vi "_GainComp_LockInAmp_2.vi"(9 "GC_LockinAmp":T3={"GPIB"="28", "wait(s)"=10.0, "measure(s) "=30.0, "save"=FALSE, "time constant"=6, "file_name"=""} {"time constant" items=["100mS"=5, "300mS"=6, "1S"=7, "3S"=8, "10S"=9]}, 10 "Control":T4={"GPIB_ATT"="28", "6501Dev#"=1, "GPIB_SP"="18", "GPIB_PM"="13", "GPIB_DSA"="11", "GPIB_DMM (TPD)"="23", "GPIB_MPI"="COM5", "mortor設定"=[{"Axis"=0, "ID"=0, "HIspeed"=200.0, "LOspeed"=100.0, "ACCEL(ms)"=100.0, "Sratio"=50.0, "フリーラン\n"=FALSE, "文字列"="DSB HOT/COLD"}, {"Axis"=1, "ID"=0, "HIspeed"=4.0, "LOspeed"=4.0, "ACCEL(ms)"=100.0, "Sratio"=50.0, "フリーラン\n"=TRUE, "文字列"="SubMM Att"}, {"Axis"=0, "ID"=0, "HIspeed"=200.0, "LOspeed"=100.0, "ACCEL(ms)"=100.0, "Sratio"=50.0, "フリーラン\n"=FALSE, "文字列"="MPI Port1"}, {"Axis"=1, "ID"=0, "HIspeed"=200.0, "LOspeed"=100.0, "ACCEL(ms)"=100.0, "Sratio"=50.0, "フリーラン\n"=FALSE, "文字列"="MPI Port2"}, {"Axis"=1, "ID"=0, "HIspeed"=200.0, "LOspeed"=100.0, "ACCEL(ms)"=100.0, "Sratio"=50.0, "フリーラン\n"=TRUE, "文字列"="gainComp"}], "DATAパス"=path "C:/Documents and Settings/band10/デスクトップ/data/cartridge/CCA03/CCA-03-13/110629_SBR_P1", "DBパス "=path "Z:/band10/Labview_ALMA/MIX95/test", "comment"="110629_SBR_P1", "ColdCarts"="003601", "Th"=299.0, "Tc"=83.0, "Set_SIS_volt"=2.1, "Offset"=0.0, "control"=0, "FreqLO"=874.0, "Set_Mag_Cur"=8.86861313868613, "MPI offset(mm)"=23.166, "HOT/COLD"=1} {"HOT/COLD" items=["DSB", "SBR (Cart.)", "GainComp", "SBR (MIX)"]; "control" items=["CLOSE LOOP", "OPEN LOOP", "Not Control"]}, 11 "Bias_LO_equip":T1={"Node address"=19, "CAN Interface"="CAN0", "Cartridge band"=10, "Slave Node in"={"Address"=19, "Serial Number"=[16, -88, -112, 75, 1, 8, 0, 24]}, "ObjHandle out"=93257792, "POL"=0, "sb"=1, "GPIB_SM (SIS S,V)"="24", "GPIB_DMM (SIS I)"="22", "GPIB_SM (MAG I) "="25", "GPIB_SG(LO)"="19", "GPIB_PW (PAMP) "="6", "GPIB_TMP1(8ch)"="12", "GPIB_TMP2(2ch)  "="13", "WCA_avg"=10, "Rsen"=10.0, "BiasModule"=1, "LOModule "=2, "WCA_LO_FREQ_SET"={"YTO Low freq. [GHz]"=14.66, "YTO High freq. [GHz]"=17.5, "Kvco"=1, "Lock Pol."=0, "SET LO FREQ"=97.111115, "Multiplier"=6.0, "YTO (HEX)"=2196, "YTO ( FREQ)"=16.18299, "NULL PLL INTEGRATOR"=FALSE}, "Res for"=0} {"Res for" items=["none", "series res", "parallel res"]; "WCA_LO_FREQ_SET"."YTO ( FREQ)" min=25 max=150 step=0.0001 format="%.3f"; "WCA_LO_FREQ_SET"."Multiplier" min=3 max=6 step=3; "WCA_LO_FREQ_SET"."SET LO FREQ" min=25 max=150 step=0.0001 format="%.3f"; "WCA_LO_FREQ_SET"."Lock Pol." items=["Lower", "Upper"]; "WCA_LO_FREQ_SET"."Kvco" items=["7.5MHz/V", "15MHz/V"]; "WCA_LO_FREQ_SET"."YTO High freq. [GHz]" format="%.3f"; "WCA_LO_FREQ_SET"."YTO Low freq. [GHz]" format="%.3f"; "LOModule" items=["Manual Gunn+PAMP"=0, "PLL GUNN+PAMP"=5, "B10Lab LO"=1, "WCA LO"=2, ""=3, "YIG発信器"=4, "none"=99]; "BiasModule" items=["B10Lab Bias"=0, "WCA BiasModule"=1, "none"=99]; "Slave Node in"."Serial Number" format="%.0x"; "Slave Node in"."Address" format="%.0x"; "Cartridge band" max=10 step=1; "Node address" format="%.0x"}) -> (3 "出力文字列":string="GainComp, 2011-02-04  14:13:24, 874.00,1, 0, 0.95,, 2.256E-3, 2.227E-3, 5.462E-6, 1.285E+0, 9.323E-1")   [LabVIEW 2017]
uses:
  <vilib>/Analysis/NI_AALBase.lvlib
panel:
  out "測定回数":dbl
  out "Ｖｃ　σ":bool
  out "Vh σ":bool
  out "Vh":bool
  out "Vc":bool
  out "TC":dbl=300.0
  out "ΔVh":dbl=4.302325581394609e-07 format="%#_6p"
  out "ΔVc":dbl=3.139534883720742e-07 format="%#_6p"
  out "GCls  2":dbl=0.08160280378442007 format="%#_6f"
  out "Error 2":dbl=0.0005369243568017377 format="%#_6f"
  out "GCdiff 2":dbl=-0.044394897546439334 format="%#_6f"
  out "Error 1":dbl=0.000518990604292761 format="%#_4f"
  out "GCls  1":dbl=0.12198673439194854 format="%#_4f"
  out "GCdiff 1":dbl=0.018739520662782047 format="%#_4f"
  out "Vh2 σ":dbl=2.8613203126074345e-06 format="%#_6p"
  out "Vh2":dbl=0.0011791627906976743 format="%#_6p"
  out "Vc2 σ":dbl=2.5850430165789864e-06 format="%#_6p"
  out "Vc2":dbl=0.0011786395348837209 format="%#_6p"
  out "AP":dbl[](array[numeric])
  out "AR":dbl[](array[numeric])
  out "AT":dbl[](array[numeric])
  out "Vh1 σ":dbl=2.507960747227626e-06 format="%#_6p"
  out "Vh1":dbl=0.0011787325581395349 format="%#_6p"
  out "Vc1 σ":dbl=1.671946233643571e-06 format="%#_6p"
  out "Vc1":dbl=0.001178953488372093 format="%#_6p"
  out "XYグラフ 2":cluster{dbl[], dbl[]}(graph)={[11.15625, 11.84375, 12.53125, 13.21875, 13.921875, 14.609375, 15.296875, 15.984375, 16.671875, 17.359375, 18.046875, 18.734375, 19.421875, 20.109375, 20.796875, 21.484375, 22.171875, 22.859375, 23.546875, 24.234375, 24.921875, 25.625, 26.3125, 27.0, 27.6875, 28.375, 29.0625, 29.75, 30.4375, 31.125, 31.8125, 32.5, 33.1875, 33.875, 34.5625, 35.25, 35.9375, 36.625, 37.3125, 38.0, 38.703125, 39.390625, 40.078125, 51.171875, 51.859375, 52.546875, 53.234375, 53.9375, 54.625, 55.3125, 56.0, 56.6875, 57.375, 58.0625, 58.75, 59.4375, 60.125, 60.8125, 61.5, 62.1875, 62.875, 63.5625, 64.25, 64.9375, 65.625, 66.328125, 67.015625, 67.703125, 68.390625, 69.078125, 69.765625, 70.453125, 71.140625, 71.828125, 72.515625, 73.203125, 73.890625, 74.578125, 75.265625, 75.953125, 76.640625, 77.328125, 78.015625, 78.71875, 79.40625, 80.09375, 91.203125, 91.890625, 92.578125, 93.265625, 93.953125, 94.640625, 95.328125, 96.015625, 96.703125, 97.390625, 98.078125, 98.765625, 99.453125, 100.140625, 100.828125, 101.515625, 102.203125, 102.890625, 103.59375, 104.28125, 104.96875, 105.65625, 106.34375, 107.03125, 107.71875, 108.40625, 109.09375, 109.78125, 110.46875, 111.15625, 111.84375, 112.53125, 113.21875, 113.90625, 114.59375, 115.28125, 115.984375, 116.671875, 117.359375, 118.046875, 118.734375, 119.421875, 120.109375, 131.203125, 131.890625, 132.578125, 133.265625, 133.953125, 134.65625, 135.34375, 136.03125, 136.71875, 137.40625, 138.09375, 138.78125, 139.46875, 140.15625, 140.84375, 141.53125, 142.21875, 142.90625, 143.59375, 144.28125, 144.96875, 145.65625, 146.34375, 147.03125, 147.734375, 148.421875, 149.109375, 149.796875, 150.484375, 151.171875, 151.859375, 152.546875, 153.234375, 153.921875, 154.609375, 155.296875, 155.984375, 156.671875, 157.359375, 158.046875, 158.734375, 159.4375, 160.125], [98.35, 97.45, 97.75, 98.25, 97.5, 97.55, 97.65, 98.1, 98.15, 98.05, 98.1, 97.95, 98.1, 98.15, 98.5, 98.6, 98.35, 97.95, 98.05, 98.4, 98.3, 98.15, 98.45, 98.0, 98.3, 97.95, 98.25, 97.85, 97.45, 97.75, 97.3, 97.1, 97.3, 97.2, 97.7, 98.1, 98.1, 97.85, 97.9, 98.15, 97.8, 97.8, 97.35, 97.9, 97.65, 98.05, 98.15, 98.05, 97.85, 97.9, 97.75, 98.3, 98.8, 98.7, 98.05, 98.2, 98.85, 97.75, 97.65, 97.85, 98.15, 98.75, 98.75, 98.2, 97.55, 97.05, 96.75, 96.45, 96.8, 97.4, 97.45, 97.75, 98.35, 98.25, 98.5, 98.9, 98.7, 98.55, 98.75, 98.25, 98.45, 98.7, 98.45, 98.1, 98.25, 98.1, 96.6, 96.95, 96.7, 96.55, 96.05, 96.3, 96.2, 96.15, 95.85, 96.7, 96.9, 97.15, 98.05, 98.0, 98.1, 97.8, 98.05, 97.95, 98.0, 98.45, 98.1, 98.25, 98.25, 98.4, 98.35, 98.2, 98.1, 97.9, 98.3, 98.45, 98.65, 98.6, 98.45, 97.95, 98.6, 98.35, 98.25, 98.25, 98.25, 98.05, 98.1, 98.45, 98.6, 98.75, 98.4, 98.3, 98.7, 99.2, 98.75, 98.35, 98.05, 97.6, 98.4, 98.45, 98.4, 98.65, 98.25, 97.8, 98.2, 98.95, 97.75, 98.4, 98.45, 98.2, 97.75, 97.75, 98.15, 97.05, 96.35, 96.2, 96.2, 96.2, 97.0, 96.5, 96.35, 96.55, 96.45, 96.95, 97.15, 97.65, 97.4, 97.45, 97.9, 97.6, 97.5, 97.5]}
  out "P":dbl=97.35 format="%#_4f"
  out "XYグラフ":cluster{dbl[], dbl[]}(graph)={[11.15625, 11.84375, 12.53125, 13.21875, 13.921875, 14.609375, 15.296875, 15.984375, 16.671875, 17.359375, 18.046875, 18.734375, 19.421875, 20.109375, 20.796875, 21.484375, 22.171875, 22.859375, 23.546875, 24.234375, 24.921875, 25.625, 26.3125, 27.0, 27.6875, 28.375, 29.0625, 29.75, 30.4375, 31.125, 31.8125, 32.5, 33.1875, 33.875, 34.5625, 35.25, 35.9375, 36.625, 37.3125, 38.0, 38.703125, 39.390625, 40.078125, 51.171875, 51.859375, 52.546875, 53.234375, 53.9375, 54.625, 55.3125, 56.0, 56.6875, 57.375, 58.0625, 58.75, 59.4375, 60.125, 60.8125, 61.5, 62.1875, 62.875, 63.5625, 64.25, 64.9375, 65.625, 66.328125, 67.015625, 67.703125, 68.390625, 69.078125, 69.765625, 70.453125, 71.140625, 71.828125, 72.515625, 73.203125, 73.890625, 74.578125, 75.265625, 75.953125, 76.640625, 77.328125, 78.015625, 78.71875, 79.40625, 80.09375, 91.203125, 91.890625, 92.578125, 93.265625, 93.953125, 94.640625, 95.328125, 96.015625, 96.703125, 97.390625, 98.078125, 98.765625, 99.453125, 100.140625, 100.828125, 101.515625, 102.203125, 102.890625, 103.59375, 104.28125, 104.96875, 105.65625, 106.34375, 107.03125, 107.71875, 108.40625, 109.09375, 109.78125, 110.46875, 111.15625, 111.84375, 112.53125, 113.21875, 113.90625, 114.59375, 115.28125, 115.984375, 116.671875, 117.359375, 118.046875, 118.734375, 119.421875, 120.109375, 131.203125, 131.890625, 132.578125, 133.265625, 133.953125, 134.65625, 135.34375, 136.03125, 136.71875, 137.40625, 138.09375, 138.78125, 139.46875, 140.15625, 140.84375, 141.53125, 142.21875, 142.90625, 143.59375, 144.28125, 144.96875, 145.65625, 146.34375, 147.03125, 147.734375, 148.421875, 149.109375, 149.796875, 150.484375, 151.171875, 151.859375, 152.546875, 153.234375, 153.921875, 154.609375, 155.296875, 155.984375, 156.671875, 157.359375, 158.046875, 158.734375, 159.4375, 160.125], [0.0011775, 0.0011775, 0.00118, 0.001182, 0.0011795, 0.001177, 0.00118, 0.001181, 0.00118, 0.00118, 0.001179, 0.0011805, 0.001179, 0.001177, 0.0011765, 0.001177, 0.0011785, 0.001181, 0.001179, 0.001178, 0.00118, 0.001176, 0.0011775, 0.001179, 0.001179, 0.0011785, 0.001179, 0.00118, 0.0011785, 0.0011795, 0.0011775, 0.00118, 0.001179, 0.001177, 0.0011785, 0.0011825, 0.0011825, 0.00118, 0.0011775, 0.001179, 0.0011755, 0.0011775, 0.0011815, 0.0011805, 0.0011795, 0.0011785, 0.00118, 0.0011825, 0.00118, 0.001174, 0.0011805, 0.001182, 0.001177, 0.00118, 0.00118, 0.00118, 0.00118, 0.001178, 0.0011815, 0.001182, 0.0011815, 0.001177, 0.001176, 0.001177, 0.001176, 0.0011765, 0.0011805, 0.001175, 0.00118, 0.0011815, 0.0011825, 0.001179, 0.0011765, 0.00118, 0.0011805, 0.00118, 0.001173, 0.0011775, 0.0011775, 0.00118, 0.001179, 0.0011735, 0.001179, 0.0011735, 0.001178, 0.001179, 0.0011835, 0.0011825, 0.001182, 0.00118, 0.0011815, 0.001181, 0.001181, 0.001175, 0.00118, 0.001179, 0.001177, 0.001184, 0.001177, 0.0011795, 0.0011815, 0.0011765, 0.001179, 0.0011835, 0.00118, 0.001178, 0.001176, 0.0011755, 0.0011785, 0.001178, 0.001176, 0.00118, 0.00118, 0.0011765, 0.0011755, 0.001178, 0.00118, 0.0011785, 0.001179, 0.001179, 0.001174, 0.001179, 0.0011725, 0.001177, 0.001177, 0.0011785, 0.0011775, 0.0011755, 0.0011785, 0.001176, 0.0011805, 0.001177, 0.0011785, 0.001178, 0.0011775, 0.0011805, 0.001178, 0.0011775, 0.001172, 0.0011745, 0.001178, 0.0011795, 0.0011815, 0.001184, 0.0011825, 0.0011795, 0.0011735, 0.0011825, 0.0011805, 0.00118, 0.0011795, 0.00118, 0.0011755, 0.001175, 0.001174, 0.001181, 0.0011825, 0.0011825, 0.00118, 0.001176, 0.001177, 0.0011805, 0.001179, 0.0011805, 0.0011825, 0.001182, 0.0011825, 0.00118, 0.0011775, 0.001181, 0.0011825, 0.0011815]}
  out "経過時間（s）":dbl=23.546875
  in  "SIS_Deflux_heater":T2={"ON開始時間（mｓ）"=3000.0, "ON継続時間（mｓ）"=1000.0, "測定終了時間（mｓ）"=60000.0, "SIS Volt（mV)"=0.5, "GPIB_PW (SISHeater) "="3", "SAVE"=TRUE}
  out "初期時間（s）":dbl=3392182452.97575
  out "R":dbl=0.002211 format="%#_6p"
  # "LO freq. [GHz]"
  # "YTO LOW\n/High Freq."
  # "ZERO Intgrtr"
  # "Node Address"
  # "Serial Number"
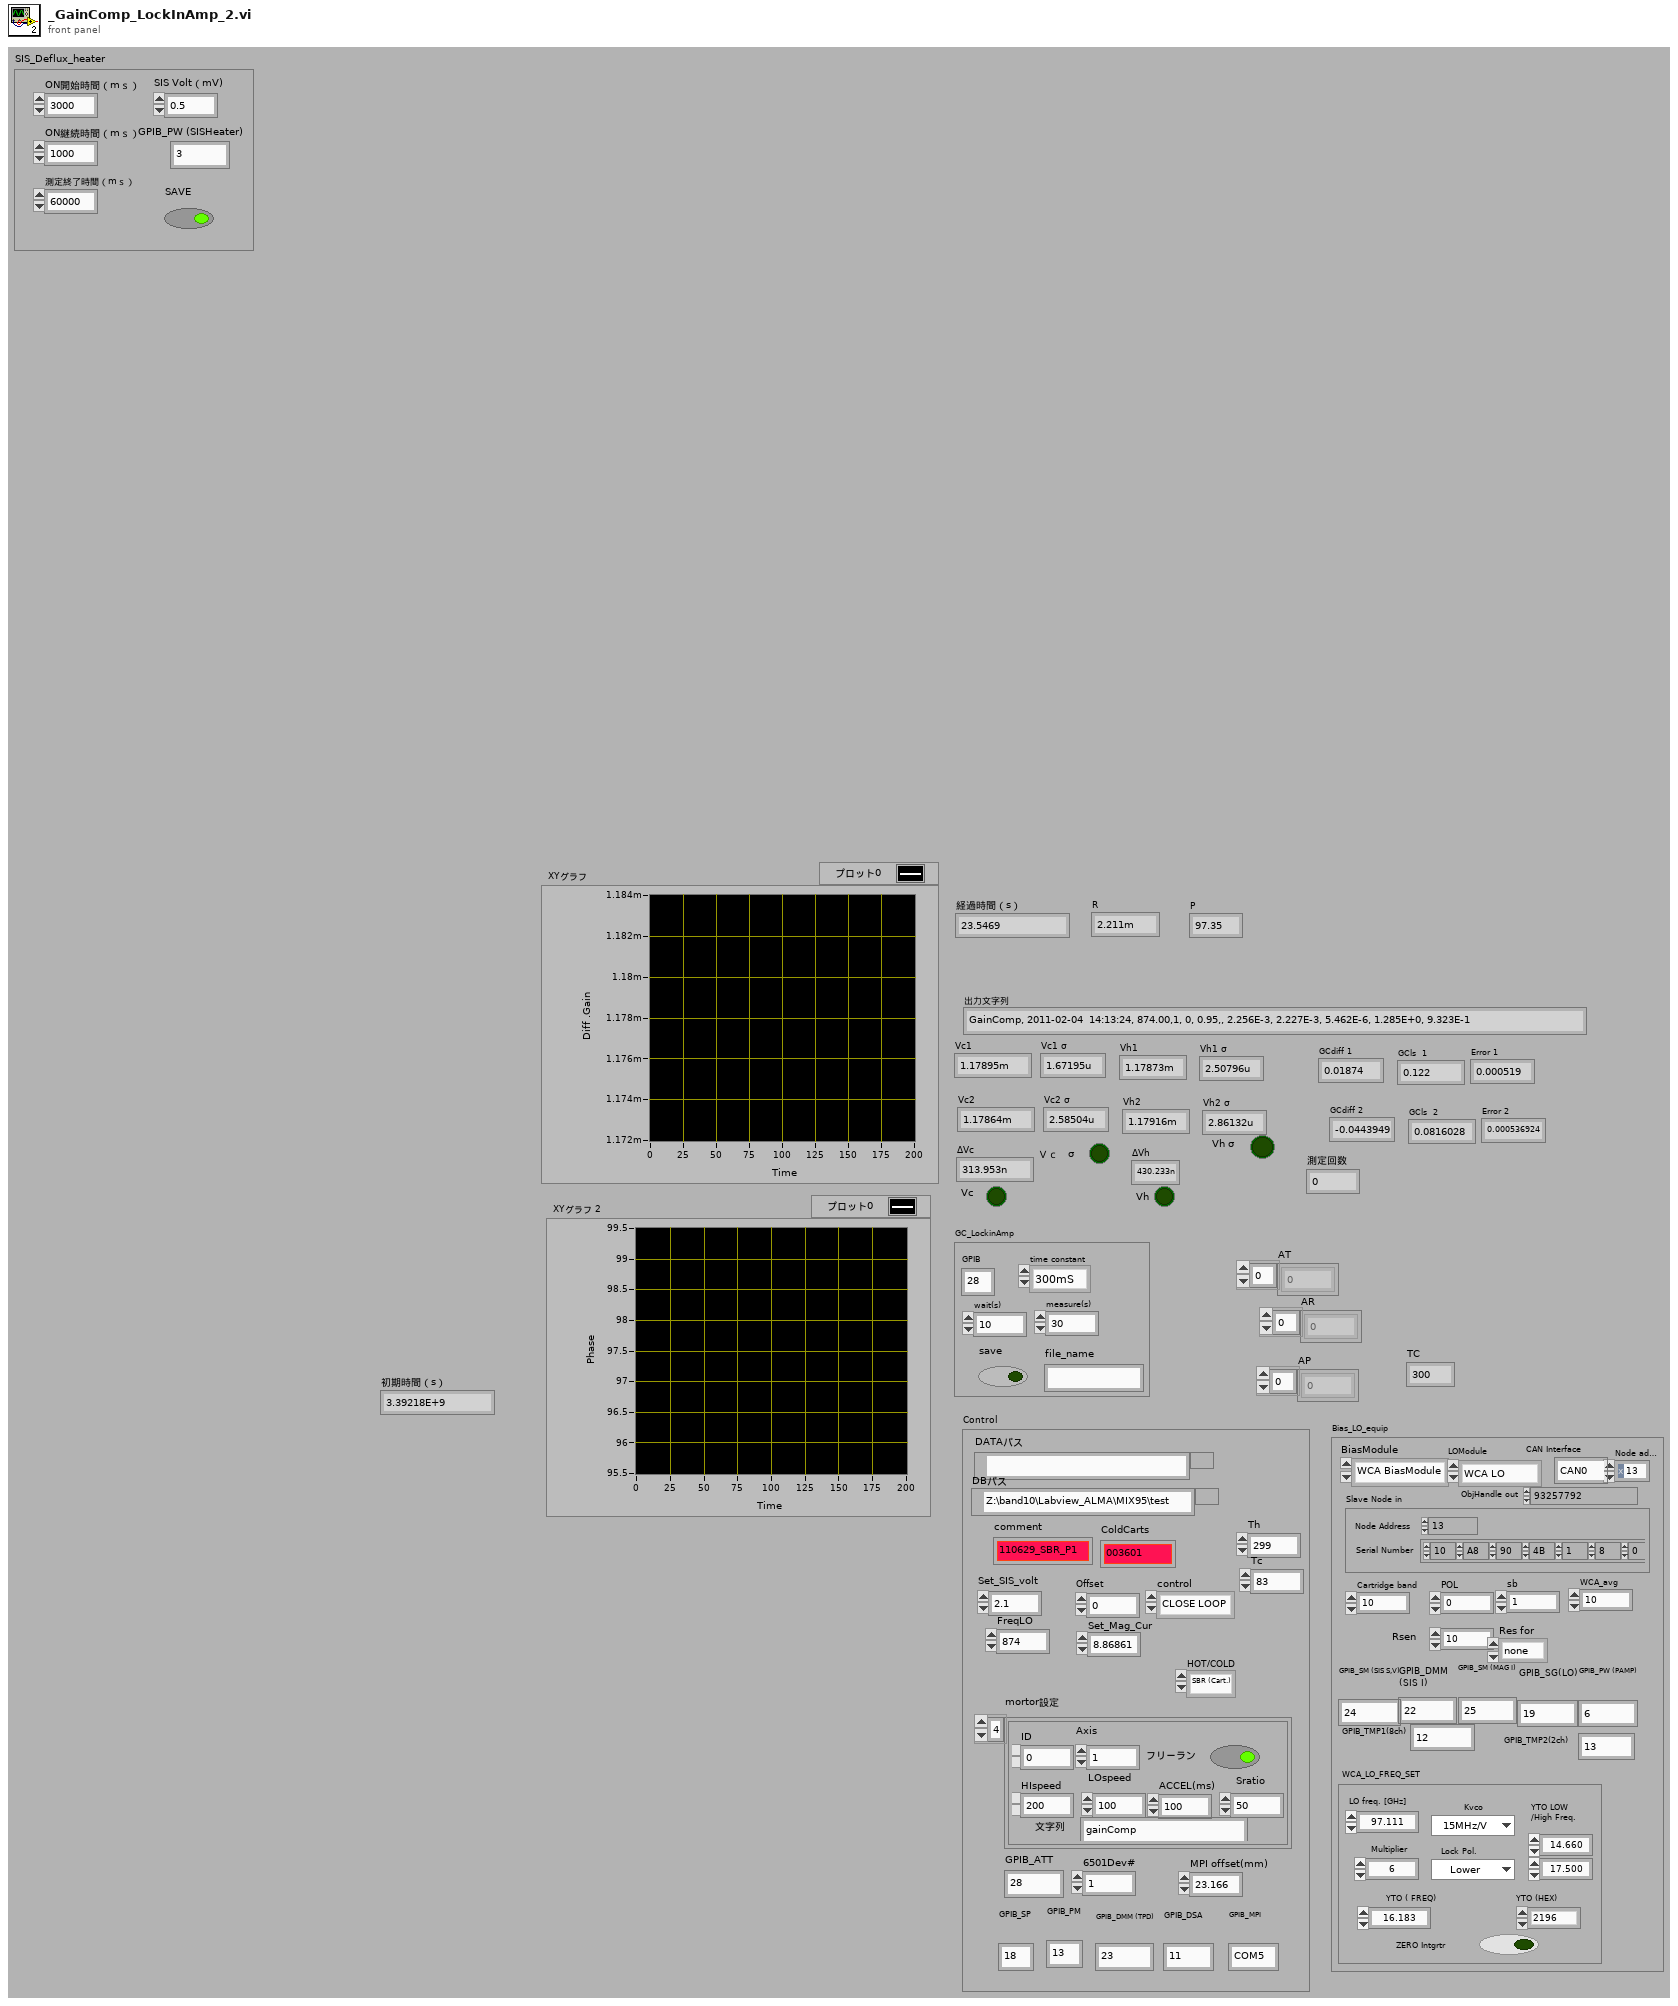
[diagram p1: front panel]
types:
  T1 = cluster{"Node address":u16, "CAN Interface":string, "Cartridge band":u32, "Slave Node in":cluster{"Address":i16, "Serial Number":i8[]}, "ObjHandle out":u32, "POL":u32, "sb":u32, "GPIB_SM (SIS S,V)":string, "GPIB_DMM (SIS I)":string, "GPIB_SM (MAG I) ":string, "GPIB_SG(LO)":string, "GPIB_PW (PAMP) ":string, "GPIB_TMP1(8ch)":string, "GPIB_TMP2(2ch)  ":string, "WCA_avg":i32, "Rsen":dbl, "BiasModule":u16, "LOModule ":u16, "WCA_LO_FREQ_SET":cluster{"YTO Low freq. [GHz]":sgl, "YTO High freq. [GHz]":sgl, "Kvco":u16, "Lock Pol.":u16, "SET LO FREQ":sgl, "Multiplier":sgl, "YTO (HEX)":u16, "YTO ( FREQ)":sgl, "NULL PLL INTEGRATOR":bool}, "Res for":u16}
  T2 = cluster{"ON開始時間（mｓ）":dbl, "ON継続時間（mｓ）":dbl, "測定終了時間（mｓ）":dbl, "SIS Volt（mV)":dbl, "GPIB_PW (SISHeater) ":string, "SAVE":bool}
  T3 = cluster{"GPIB":string, "wait(s)":dbl, "measure(s) ":dbl, "save":bool, "time constant":u16, "file_name":string}
  T4 = cluster{"GPIB_ATT":string, "6501Dev#":i16, "GPIB_SP":string, "GPIB_PM":string, "GPIB_DSA":string, "GPIB_DMM (TPD)":string, "GPIB_MPI":string, "mortor設定":cluster{"Axis":i16, "ID":i16, "HIspeed":dbl, "LOspeed":dbl, "ACCEL(ms)":dbl, "Sratio":dbl, "フリーラン\n":bool, "文字列":string}[], "DATAパス":path, "DBパス ":path, "comment":string, "ColdCarts":string, "Th":dbl, "Tc":dbl, "Set_SIS_volt":dbl, "Offset":dbl, "control":u16, "FreqLO":dbl, "Set_Mag_Cur":dbl, "MPI offset(mm)":dbl, "HOT/COLD":u16}
  T5 = cluster{"Axis":i16, "ID":i16, "HIspeed":dbl, "LOspeed":dbl, "ACCEL(ms)":dbl, "Sratio":dbl, "フリーラン\n":bool, "文字列":string}[]
  T6 = cluster{"Axis":i16, "ID":i16, "HIspeed":dbl, "LOspeed":dbl, "ACCEL(ms)":dbl, "Sratio":dbl, "フリーラン\n":bool, "文字列":string}
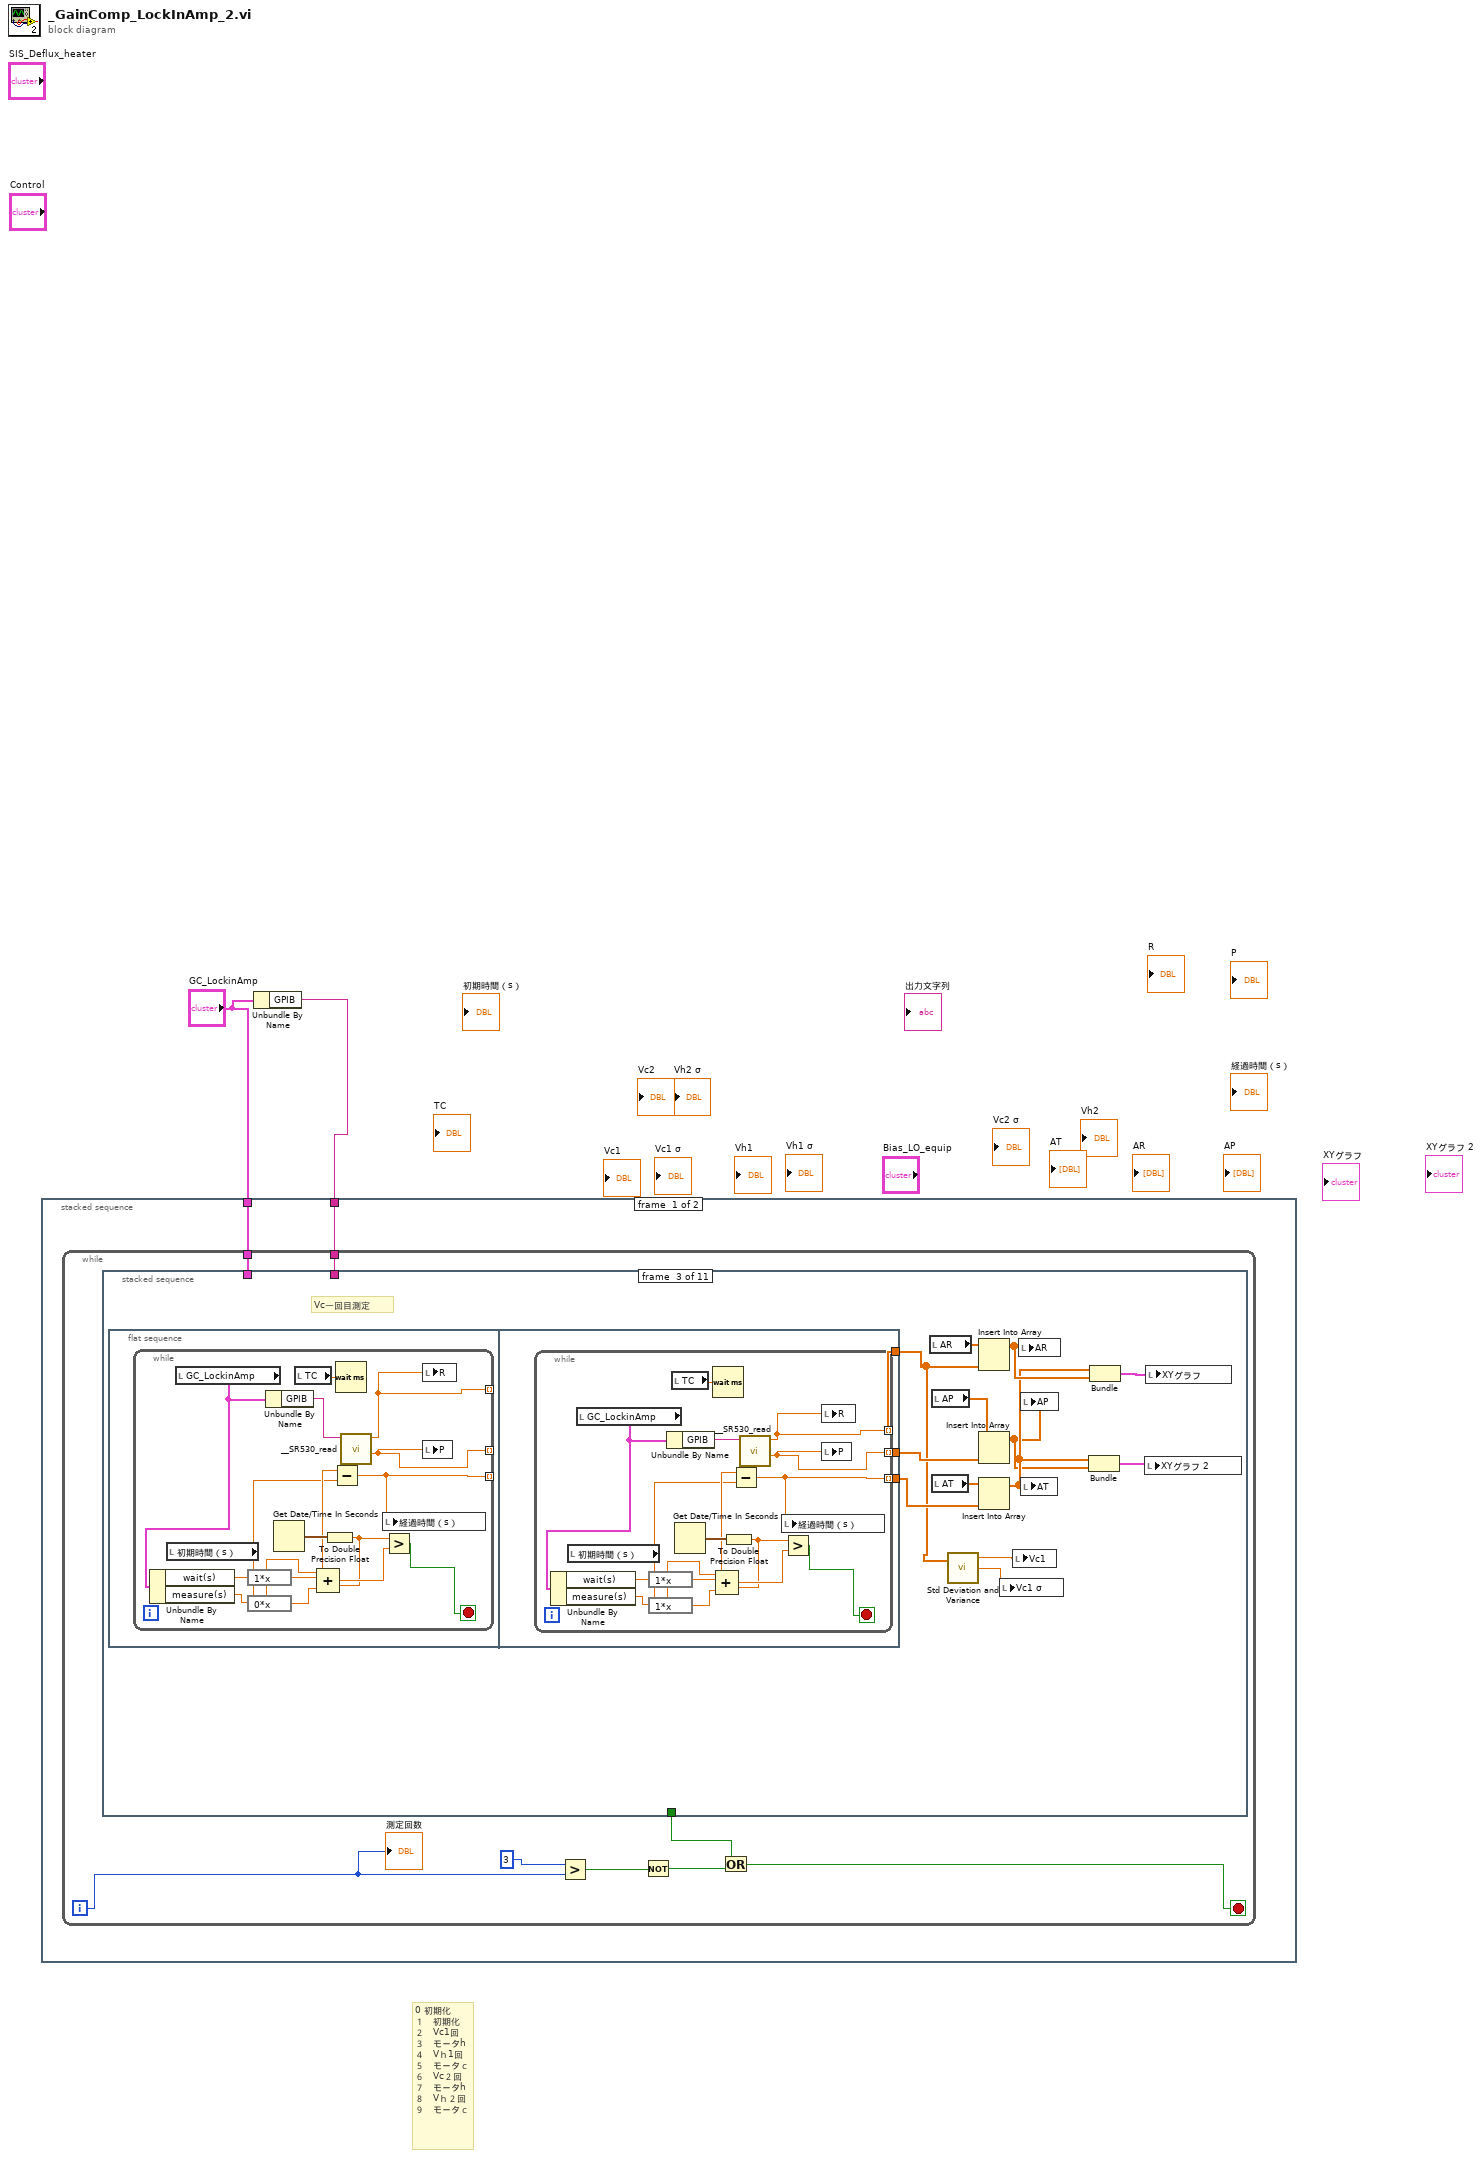
[diagram p0: block diagram]
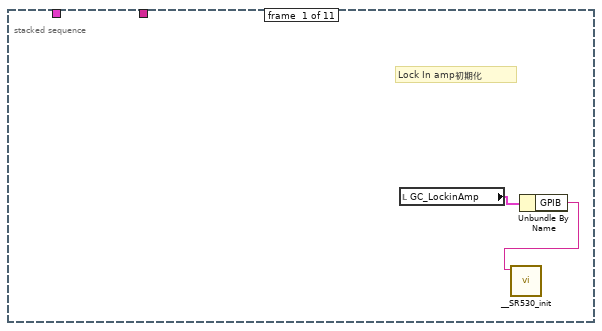
[diagram p2: hidden frame]
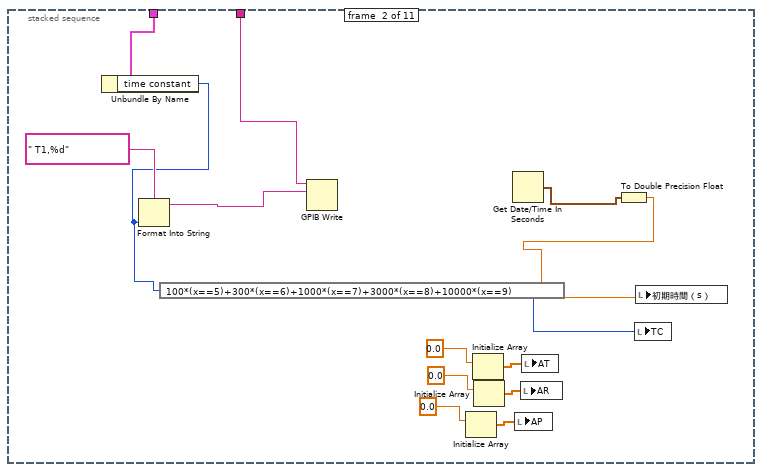
[diagram p3: hidden frame]
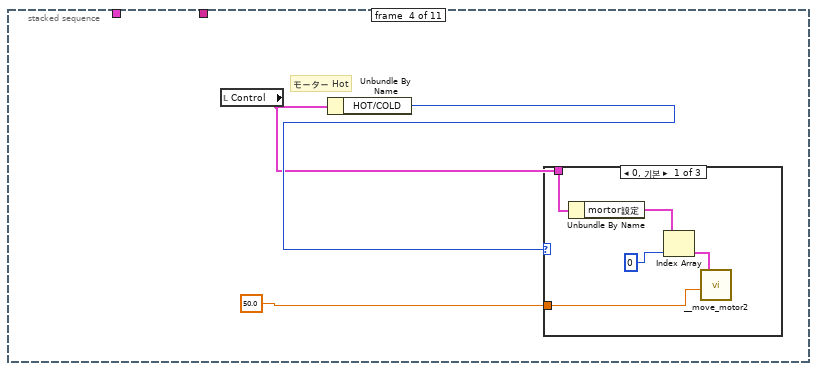
[diagram p4: hidden frame]
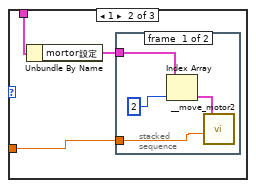
[diagram p5: hidden frame]
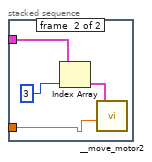
[diagram p6: hidden frame]
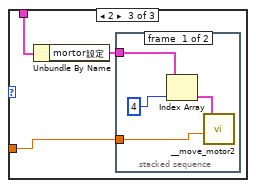
[diagram p7: hidden frame]
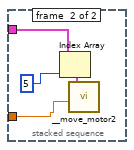
[diagram p8: hidden frame]
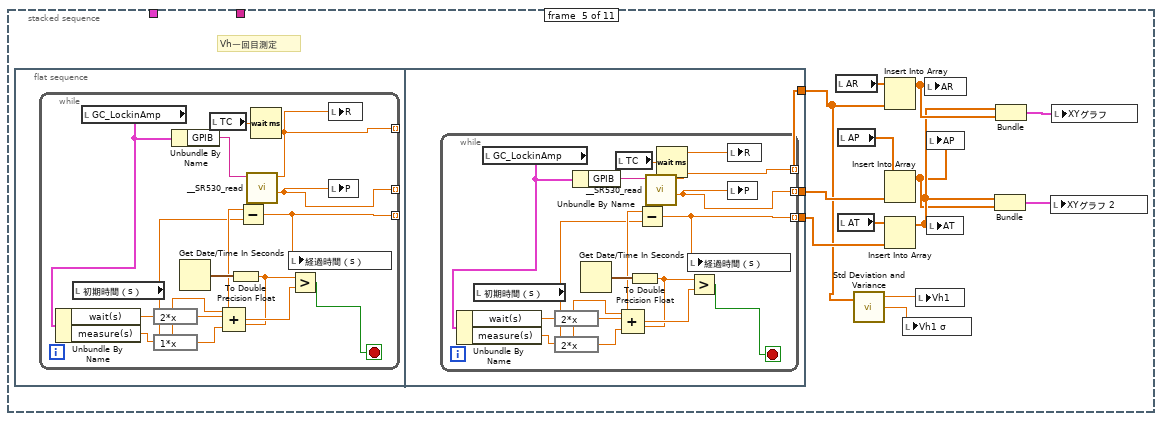
[diagram p9: hidden frame]
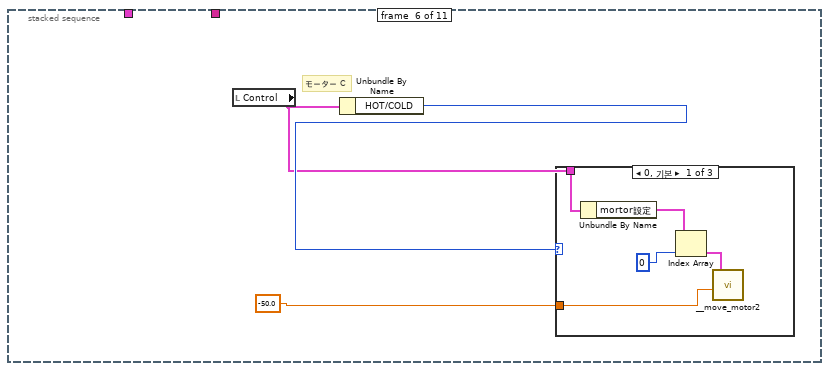
[diagram p10: hidden frame]
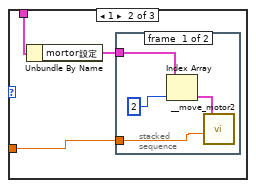
[diagram p11: hidden frame]
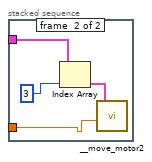
[diagram p12: hidden frame]
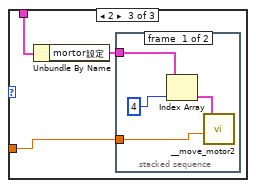
[diagram p13: hidden frame]
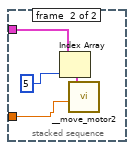
[diagram p14: hidden frame]
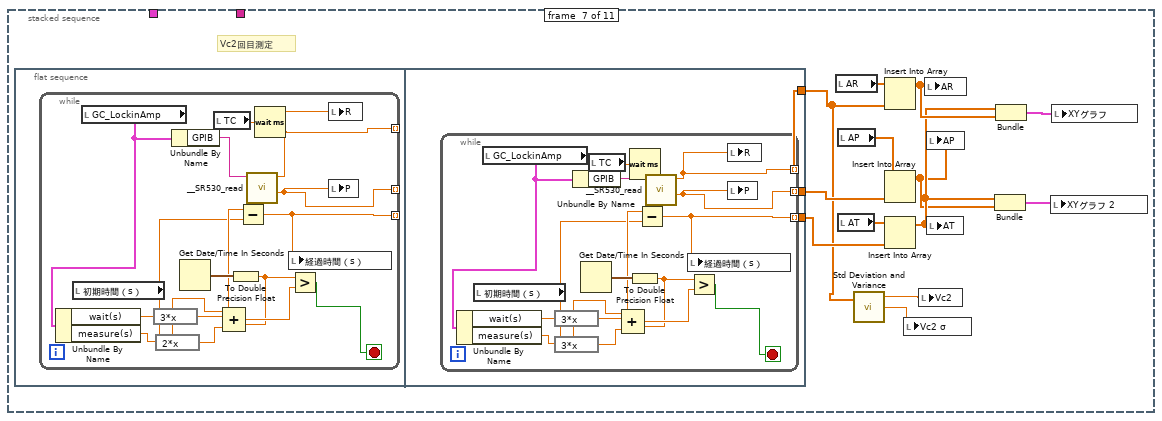
[diagram p15: hidden frame]
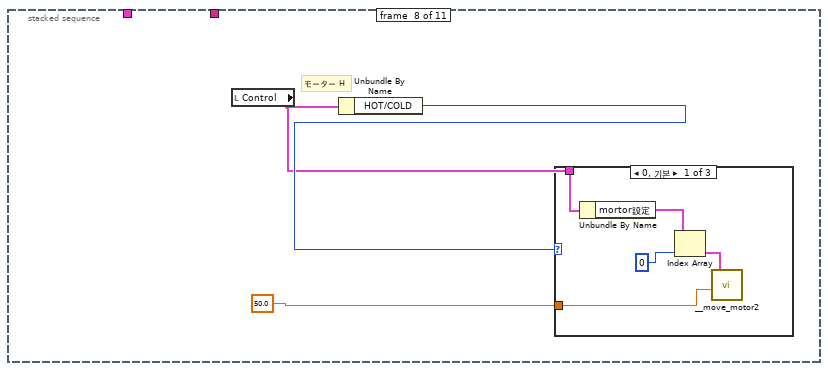
[diagram p16: hidden frame]
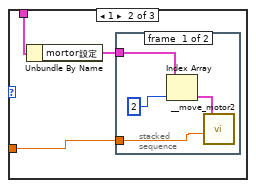
[diagram p17: hidden frame]
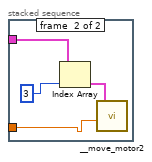
[diagram p18: hidden frame]
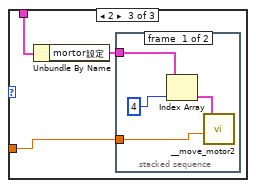
[diagram p19: hidden frame]
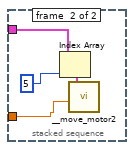
[diagram p20: hidden frame]
diagram:
  # "0 初期化\n１　初期化\n２　Vc1回\n３　モータh\n４　Vｈ1回\n５　モータｃ\n６　Vc２回\n７　モータh\n８　Vｈ２回\n９　モータｃ"
  n1 = Unbundle By Name("GC_LockinAmp") -> ("GPIB"=w2:string)
  n2 = stacked-sequence {
    tunnel: w2 -> [w4 _]
    tunnel: "GC_LockinAmp" -> [w3 _]
    frame #0 {
      n3 = while {
        tunnel: w4 -> [w12]
        tunnel: w3 -> [w11]
        i -> [w5]
        stop <- w7 stop-if-true
        n4 = stacked-sequence {
          tunnel: w12 -> [_ w20 _ _ _ _ _ _ _ _ _]
          tunnel: w11 -> [_ w19 _ _ _ _ _ _ _ _ _]
          tunnel: [_ _ _ _ _ _ _ _ _ _ w338] -> w9
          frame #0 {
            # "Lock In amp初期化"
            n5 = local read "GC_LockinAmp"() -> (w14:T3)
            n6 = Unbundle By Name(w14) -> ("GPIB"=w13:string)
            n7 = call "__SR530_init.vi"("GPIB"=w13) -> ()  [unwired: 7 in]
          }
          frame #1 {
            n8 = Unbundle By Name(w19) -> ("time constant"=w16:u16)
            n9 = Format Into String(format string=" T1,%d", w16) -> (resulting string=w17:string)  [unwired: 2 in, 1 out]
            n10 = expression code="100*(x==5)+300*(x==6)+1000*(x==7)+3000*(x==8)+10000*(x==9)"(w16) -> (w15:u16)
            n11 = GPIB Write(0:w20, 1:w17) -> ()  [unwired: 3 in, 2 out]
            n12 = Initialize Array(0.0) -> (w22:dbl[])  [unwired: 1 in]
            n13 = Initialize Array(0.0) -> (w26:dbl[])  [unwired: 1 in]
            n14 = Initialize Array(0.0) -> (w23:dbl[])  [unwired: 1 in]
            n15 = Get Date/Time In Seconds() -> (seconds since 1Jan1904=w28:timestamp)
            n16 = local write "AP"(w22) -> ()
            n17 = local write "AR"(w23) -> ()
            n18 = local write "AT"(w26) -> ()
            n19 = To Double Precision Float(number=w28) -> (double precision float=w27:dbl)
            n20 = local write "TC"(w15) -> ()
            n21 = local write "初期時間（s）"(w27) -> ()
          }
          frame #2 {
            # "Vc一回目測定"
            n22 = flat-sequence {
              tunnel: [w59] -> w38
              tunnel: [w58] -> w34
              tunnel: [w57] -> w35
              frame #0 {
                n23 = while {
                  tunnel: [w47] -> _ mode=indexing
                  tunnel: [w46] -> _ mode=indexing
                  tunnel: [w45] -> _ mode=indexing
                  stop <- w50 stop-if-true
                  n24 = local read "初期時間（s）"() -> (w48:dbl)
                  n25 = local read "GC_LockinAmp"() -> (w44:T3)
                  n26 = Unbundle By Name(w44) -> ("wait(s)"=w55:dbl, "measure(s)"=w54:dbl)
                  n27 = expression code="1*x"(w55) -> (w53:dbl)
                  n28 = expression code="0*x"(w54) -> (w51:dbl)
                  n29 = Unbundle By Name(w44) -> ("GPIB"=w43:string)
                  n30 = Get Date/Time In Seconds() -> (seconds since 1Jan1904=w56:timestamp)
                  n31 = local read "TC"() -> (w42:dbl)
                  n32 = Compound Arithmetic op=ADD(w48, w53, w51) -> (w52:dbl)
                  n33 = To Double Precision Float(number=w56) -> (double precision float=w49:dbl)
                  n34 = Subtract(x=w49, y=w48) -> (x-y=w46:dbl)
                  n35 = Wait (ms)(milliseconds to wait=w42) -> ()  [unwired: 1 out]
                  n36 = call "__SR530_read.vi"("GPIB"=w43) -> ("Phase"=w45:dbl, "R"=w47:dbl)  [unwired: 5 in]
                  n37 = local write "経過時間（s）"(w46) -> ()
                  n38 = Greater?(x=w49, y=w52) -> (0:w50:bool)
                  n39 = local write "R"(w47) -> ()
                  n40 = local write "P"(w45) -> ()
                }
              }
              frame #1 {
                n41 = while {
                  tunnel: [w65] -> w58 mode=indexing
                  tunnel: [w64] -> w59 mode=indexing
                  tunnel: [w63] -> w57 mode=indexing
                  stop <- w68 stop-if-true
                  n42 = local read "初期時間（s）"() -> (w66:dbl)
                  n43 = local read "GC_LockinAmp"() -> (w62:T3)
                  n44 = Unbundle By Name(w62) -> ("wait(s)"=w73:dbl, "measure(s)"=w72:dbl)
                  n45 = expression code="1*x"(w73) -> (w71:dbl)
                  n46 = expression code="1*x"(w72) -> (w69:dbl)
                  n47 = Unbundle By Name(w62) -> ("GPIB"=w61:string)
                  n48 = local read "TC"() -> (w60:dbl)
                  n49 = Get Date/Time In Seconds() -> (seconds since 1Jan1904=w74:timestamp)
                  n50 = Wait (ms)(milliseconds to wait=w60) -> ()  [unwired: 1 out]
                  n51 = Compound Arithmetic op=ADD(w66, w71, w69) -> (w70:dbl)
                  n52 = To Double Precision Float(number=w74) -> (double precision float=w67:dbl)
                  n53 = Subtract(x=w67, y=w66) -> (x-y=w64:dbl)
                  n54 = call "__SR530_read.vi"("GPIB"=w61) -> ("Phase"=w63:dbl, "R"=w65:dbl)  [unwired: 5 in]
                  n55 = local write "経過時間（s）"(w64) -> ()
                  n56 = Greater?(x=w67, y=w70) -> (0:w68:bool)
                  n57 = local write "R"(w65) -> ()
                  n58 = local write "P"(w63) -> ()
                }
              }
            }
            n59 = local read "AR"() -> (w36:dbl[])
            n60 = local read "AP"() -> (w37:dbl[])
            n61 = local read "AT"() -> (w39:dbl[])
            n62 = call <vilib>:"Std Deviation and Variance.vi"("X"=w34) -> ("mean"=w41:dbl, "standard deviation"=w40:dbl)  [unwired: 1 in, 1 out]
            n63 = Insert Into Array(array=w36, new element=w34) -> (w33:dbl[])  [unwired: 1 in]
            n64 = Insert Into Array(array=w37, new element=w35) -> (w31:dbl[])  [unwired: 1 in]
            n65 = Insert Into Array(array=w39, new element=w38) -> (w32:dbl[])  [unwired: 1 in]
            n66 = local write "Vc1 σ"(w40) -> ()
            n67 = local write "Vc1"(w41) -> ()
            n68 = local write "AR"(w33) -> ()
            n69 = local write "AP"(w31) -> ()
            n70 = local write "AT"(w32) -> ()
            n71 = Bundle("AT"=w32, "AP"=w31) -> (w30:cluster{"AT":dbl[], "AP":dbl[]})  [unwired: 1 in]
            n72 = Bundle("AT"=w32, "AR"=w33) -> (w29:cluster{"AT":dbl[], "AR ":dbl[]})  [unwired: 1 in]
            n73 = local write "XYグラフ 2"(w30) -> ()
            n74 = local write "XYグラフ"(w29) -> ()
          }
          frame #3 {
            # "モーター Hot"
            n75 = local read "Control"() -> (w75:T4)
            n76 = Unbundle By Name(w75) -> ("HOT/COLD"=w76:u16)
            n77 = case shown="0, 기본" w76 {
              tunnel: w75 -> [w81 w85 w96]
              tunnel: 50.0 -> [w78 w83 w94]
              frame 0, Default {
                n78 = Unbundle By Name(w81) -> ("mortor設定"=w80:T5)
                n79 = Index Array(array=w80, index=0) -> (element=w79:T6)
                n80 = call "__move_motor2.vi"("Moving distance"=w78, "motor setup"=w79) -> ()  [unwired: 2 in, 2 out]
              }
              frame 1 {
                n81 = Unbundle By Name(w85) -> ("mortor設定"=w84:T5)
                n82 = stacked-sequence {
                  tunnel: w84 -> [w88 w92]
                  tunnel: w83 -> [w86 w90]
                  frame #0 {
                    n83 = Index Array(array=w88, index=2) -> (element=w87:T6)
                    n84 = call "__move_motor2.vi"("Moving distance"=w86, "motor setup"=w87) -> ()  [unwired: 2 in, 2 out]
                  }
                  frame #1 {
                    n85 = Index Array(array=w92, index=3) -> (element=w91:T6)
                    n86 = call "__move_motor2.vi"("Moving distance"=w90, "motor setup"=w91) -> ()  [unwired: 2 in, 2 out]
                  }
                }
              }
              frame 2 {
                n87 = Unbundle By Name(w96) -> ("mortor設定"=w95:T5)
                n88 = stacked-sequence {
                  tunnel: w95 -> [w99 w103]
                  tunnel: w94 -> [w97 w101]
                  frame #0 {
                    n89 = Index Array(array=w99, index=4) -> (element=w98:T6)
                    n90 = call "__move_motor2.vi"("Moving distance"=w97, "motor setup"=w98) -> ()  [unwired: 2 in, 2 out]
                  }
                  frame #1 {
                    n91 = Index Array(array=w103, index=5) -> (element=w102:T6)
                    n92 = call "__move_motor2.vi"("Moving distance"=w101, "motor setup"=w102) -> ()  [unwired: 2 in, 2 out]
                  }
                }
              }
            }
          }
          frame #4 {
            # "Vh一回目測定"
            n93 = flat-sequence {
              tunnel: [w135] -> w114
              tunnel: [w134] -> w110
              tunnel: [w133] -> w111
              frame #0 {
                n94 = while {
                  tunnel: [w123] -> _ mode=indexing
                  tunnel: [w122] -> _ mode=indexing
                  tunnel: [w121] -> _ mode=indexing
                  stop <- w126 stop-if-true
                  n95 = local read "初期時間（s）"() -> (w124:dbl)
                  n96 = local read "GC_LockinAmp"() -> (w120:T3)
                  n97 = Unbundle By Name(w120) -> ("wait(s)"=w131:dbl, "measure(s)"=w130:dbl)
                  n98 = expression code="2*x"(w131) -> (w129:dbl)
                  n99 = expression code="1*x"(w130) -> (w127:dbl)
                  n100 = Unbundle By Name(w120) -> ("GPIB"=w119:string)
                  n101 = Get Date/Time In Seconds() -> (seconds since 1Jan1904=w132:timestamp)
                  n102 = local read "TC"() -> (w118:dbl)
                  n103 = Compound Arithmetic op=ADD(w124, w129, w127) -> (w128:dbl)
                  n104 = To Double Precision Float(number=w132) -> (double precision float=w125:dbl)
                  n105 = Subtract(x=w125, y=w124) -> (x-y=w122:dbl)
                  n106 = call "__SR530_read.vi"("GPIB"=w119) -> ("Phase"=w121:dbl, "R"=w123:dbl)  [unwired: 5 in]
                  n107 = Wait (ms)(milliseconds to wait=w118) -> ()  [unwired: 1 out]
                  n108 = local write "経過時間（s）"(w122) -> ()
                  n109 = Greater?(x=w125, y=w128) -> (0:w126:bool)
                  n110 = local write "R"(w123) -> ()
                  n111 = local write "P"(w121) -> ()
                }
              }
              frame #1 {
                n112 = while {
                  tunnel: [w141] -> w134 mode=indexing
                  tunnel: [w140] -> w135 mode=indexing
                  tunnel: [w139] -> w133 mode=indexing
                  stop <- w144 stop-if-true
                  n113 = local read "初期時間（s）"() -> (w142:dbl)
                  n114 = local read "GC_LockinAmp"() -> (w138:T3)
                  n115 = Unbundle By Name(w138) -> ("wait(s)"=w149:dbl, "measure(s)"=w148:dbl)
                  n116 = expression code="2*x"(w149) -> (w147:dbl)
                  n117 = expression code="2*x"(w148) -> (w145:dbl)
                  n118 = Unbundle By Name(w138) -> ("GPIB"=w137:string)
                  n119 = Get Date/Time In Seconds() -> (seconds since 1Jan1904=w150:timestamp)
                  n120 = local read "TC"() -> (w136:dbl)
                  n121 = Compound Arithmetic op=ADD(w142, w147, w145) -> (w146:dbl)
                  n122 = To Double Precision Float(number=w150) -> (double precision float=w143:dbl)
                  n123 = Subtract(x=w143, y=w142) -> (x-y=w140:dbl)
                  n124 = call "__SR530_read.vi"("GPIB"=w137) -> ("Phase"=w139:dbl, "R"=w141:dbl)  [unwired: 5 in]
                  n125 = Wait (ms)(milliseconds to wait=w136) -> ()  [unwired: 1 out]
                  n126 = local write "経過時間（s）"(w140) -> ()
                  n127 = Greater?(x=w143, y=w146) -> (0:w144:bool)
                  n128 = local write "R"(w141) -> ()
                  n129 = local write "P"(w139) -> ()
                }
              }
            }
            n130 = local read "AR"() -> (w112:dbl[])
            n131 = local read "AP"() -> (w113:dbl[])
            n132 = local read "AT"() -> (w115:dbl[])
            n133 = call <vilib>:"Std Deviation and Variance.vi"("X"=w110) -> ("mean"=w117:dbl, "standard deviation"=w116:dbl)  [unwired: 1 in, 1 out]
            n134 = Insert Into Array(array=w112, new element=w110) -> (w109:dbl[])  [unwired: 1 in]
            n135 = Insert Into Array(array=w113, new element=w111) -> (w107:dbl[])  [unwired: 1 in]
            n136 = Insert Into Array(array=w115, new element=w114) -> (w108:dbl[])  [unwired: 1 in]
            n137 = local write "Vh1 σ"(w116) -> ()
            n138 = local write "Vh1"(w117) -> ()
            n139 = local write "AR"(w109) -> ()
            n140 = local write "AP"(w107) -> ()
            n141 = local write "AT"(w108) -> ()
            n142 = Bundle("AT"=w108, "AP"=w107) -> (w106:cluster{"AT":dbl[], "AP":dbl[]})  [unwired: 1 in]
            n143 = Bundle("AT"=w108, "AR"=w109) -> (w105:cluster{"AT":dbl[], "AR ":dbl[]})  [unwired: 1 in]
            n144 = local write "XYグラフ 2"(w106) -> ()
            n145 = local write "XYグラフ"(w105) -> ()
          }
          frame #5 {
            # "モーター C"
            n146 = local read "Control"() -> (w151:T4)
            n147 = Unbundle By Name(w151) -> ("HOT/COLD"=w152:u16)
            n148 = case shown="0, 기본" w152 {
              tunnel: w151 -> [w157 w161 w172]
              tunnel: -50.0 -> [w154 w159 w170]
              frame 0, Default {
                n149 = Unbundle By Name(w157) -> ("mortor設定"=w156:T5)
                n150 = Index Array(array=w156, index=0) -> (element=w155:T6)
                n151 = call "__move_motor2.vi"("Moving distance"=w154, "motor setup"=w155) -> ()  [unwired: 2 in, 2 out]
              }
              frame 1 {
                n152 = Unbundle By Name(w161) -> ("mortor設定"=w160:T5)
                n153 = stacked-sequence {
                  tunnel: w160 -> [w164 w168]
                  tunnel: w159 -> [w162 w166]
                  frame #0 {
                    n154 = Index Array(array=w164, index=2) -> (element=w163:T6)
                    n155 = call "__move_motor2.vi"("Moving distance"=w162, "motor setup"=w163) -> ()  [unwired: 2 in, 2 out]
                  }
                  frame #1 {
                    n156 = Index Array(array=w168, index=3) -> (element=w167:T6)
                    n157 = call "__move_motor2.vi"("Moving distance"=w166, "motor setup"=w167) -> ()  [unwired: 2 in, 2 out]
                  }
                }
              }
              frame 2 {
                n158 = Unbundle By Name(w172) -> ("mortor設定"=w171:T5)
                n159 = stacked-sequence {
                  tunnel: w171 -> [w175 w179]
                  tunnel: w170 -> [w173 w177]
                  frame #0 {
                    n160 = Index Array(array=w175, index=4) -> (element=w174:T6)
                    n161 = call "__move_motor2.vi"("Moving distance"=w173, "motor setup"=w174) -> ()  [unwired: 2 in, 2 out]
                  }
                  frame #1 {
                    n162 = Index Array(array=w179, index=5) -> (element=w178:T6)
                    n163 = call "__move_motor2.vi"("Moving distance"=w177, "motor setup"=w178) -> ()  [unwired: 2 in, 2 out]
                  }
                }
              }
            }
          }
          frame #6 {
            # "Vc2回目測定"
            n164 = flat-sequence {
              tunnel: [w211] -> w190
              tunnel: [w210] -> w186
              tunnel: [w209] -> w187
              frame #0 {
                n165 = while {
                  tunnel: [w199] -> _ mode=indexing
                  tunnel: [w198] -> _ mode=indexing
                  tunnel: [w197] -> _ mode=indexing
                  stop <- w202 stop-if-true
                  n166 = local read "初期時間（s）"() -> (w200:dbl)
                  n167 = local read "GC_LockinAmp"() -> (w196:T3)
                  n168 = Unbundle By Name(w196) -> ("wait(s)"=w207:dbl, "measure(s)"=w206:dbl)
                  n169 = expression code="3*x"(w207) -> (w205:dbl)
                  n170 = expression code="2*x"(w206) -> (w203:dbl)
                  n171 = Unbundle By Name(w196) -> ("GPIB"=w195:string)
                  n172 = Get Date/Time In Seconds() -> (seconds since 1Jan1904=w208:timestamp)
                  n173 = local read "TC"() -> (w194:dbl)
                  n174 = Compound Arithmetic op=ADD(w200, w205, w203) -> (w204:dbl)
                  n175 = To Double Precision Float(number=w208) -> (double precision float=w201:dbl)
                  n176 = Subtract(x=w201, y=w200) -> (x-y=w198:dbl)
                  n177 = call "__SR530_read.vi"("GPIB"=w195) -> ("Phase"=w197:dbl, "R"=w199:dbl)  [unwired: 5 in]
                  n178 = Wait (ms)(milliseconds to wait=w194) -> ()  [unwired: 1 out]
                  n179 = local write "経過時間（s）"(w198) -> ()
                  n180 = Greater?(x=w201, y=w204) -> (0:w202:bool)
                  n181 = local write "R"(w199) -> ()
                  n182 = local write "P"(w197) -> ()
                }
              }
              frame #1 {
                n183 = while {
                  tunnel: [w217] -> w210 mode=indexing
                  tunnel: [w216] -> w211 mode=indexing
                  tunnel: [w215] -> w209 mode=indexing
                  stop <- w220 stop-if-true
                  n184 = local read "初期時間（s）"() -> (w218:dbl)
                  n185 = local read "GC_LockinAmp"() -> (w214:T3)
                  n186 = Unbundle By Name(w214) -> ("wait(s)"=w225:dbl, "measure(s)"=w224:dbl)
                  n187 = expression code="3*x"(w225) -> (w223:dbl)
                  n188 = expression code="3*x"(w224) -> (w221:dbl)
                  n189 = Unbundle By Name(w214) -> ("GPIB"=w213:string)
                  n190 = Get Date/Time In Seconds() -> (seconds since 1Jan1904=w226:timestamp)
                  n191 = local read "TC"() -> (w212:dbl)
                  n192 = Compound Arithmetic op=ADD(w218, w223, w221) -> (w222:dbl)
                  n193 = Wait (ms)(milliseconds to wait=w212) -> ()  [unwired: 1 out]
                  n194 = To Double Precision Float(number=w226) -> (double precision float=w219:dbl)
                  n195 = Subtract(x=w219, y=w218) -> (x-y=w216:dbl)
                  n196 = call "__SR530_read.vi"("GPIB"=w213) -> ("Phase"=w215:dbl, "R"=w217:dbl)  [unwired: 5 in]
                  n197 = local write "経過時間（s）"(w216) -> ()
                  n198 = Greater?(x=w219, y=w222) -> (0:w220:bool)
                  n199 = local write "R"(w217) -> ()
                  n200 = local write "P"(w215) -> ()
                }
              }
            }
            n201 = local read "AR"() -> (w188:dbl[])
            n202 = local read "AP"() -> (w189:dbl[])
            n203 = local read "AT"() -> (w191:dbl[])
            n204 = call <vilib>:"Std Deviation and Variance.vi"("X"=w186) -> ("mean"=w193:dbl, "standard deviation"=w192:dbl)  [unwired: 1 in, 1 out]
            n205 = Insert Into Array(array=w188, new element=w186) -> (w185:dbl[])  [unwired: 1 in]
            n206 = Insert Into Array(array=w189, new element=w187) -> (w183:dbl[])  [unwired: 1 in]
            n207 = Insert Into Array(array=w191, new element=w190) -> (w184:dbl[])  [unwired: 1 in]
            n208 = local write "Vc2 σ"(w192) -> ()
            n209 = local write "Vc2"(w193) -> ()
            n210 = local write "AR"(w185) -> ()
            n211 = local write "AP"(w183) -> ()
            n212 = local write "AT"(w184) -> ()
            n213 = Bundle("AT"=w184, "AP"=w183) -> (w182:cluster{"AT":dbl[], "AP":dbl[]})  [unwired: 1 in]
            n214 = Bundle("AT"=w184, "AR"=w185) -> (w181:cluster{"AT":dbl[], "AR ":dbl[]})  [unwired: 1 in]
            n215 = local write "XYグラフ 2"(w182) -> ()
            n216 = local write "XYグラフ"(w181) -> ()
          }
          frame #7 {
            # "モーター H"
            n217 = local read "Control"() -> (w227:T4)
            n218 = Unbundle By Name(w227) -> ("HOT/COLD"=w228:u16)
            n219 = case shown="0, 기본" w228 {
              tunnel: w227 -> [w233 w237 w248]
              tunnel: 50.0 -> [w230 w235 w246]
              frame 0, Default {
                n220 = Unbundle By Name(w233) -> ("mortor設定"=w232:T5)
                n221 = Index Array(array=w232, index=0) -> (element=w231:T6)
                n222 = call "__move_motor2.vi"("Moving distance"=w230, "motor setup"=w231) -> ()  [unwired: 2 in, 2 out]
              }
              frame 1 {
                n223 = Unbundle By Name(w237) -> ("mortor設定"=w236:T5)
                n224 = stacked-sequence {
                  tunnel: w236 -> [w240 w244]
                  tunnel: w235 -> [w238 w242]
                  frame #0 {
                    n225 = Index Array(array=w240, index=2) -> (element=w239:T6)
                    n226 = call "__move_motor2.vi"("Moving distance"=w238, "motor setup"=w239) -> ()  [unwired: 2 in, 2 out]
                  }
                  frame #1 {
                    n227 = Index Array(array=w244, index=3) -> (element=w243:T6)
                    n228 = call "__move_motor2.vi"("Moving distance"=w242, "motor setup"=w243) -> ()  [unwired: 2 in, 2 out]
                  }
                }
              }
              frame 2 {
                n229 = Unbundle By Name(w248) -> ("mortor設定"=w247:T5)
                n230 = stacked-sequence {
                  tunnel: w247 -> [w251 w255]
                  tunnel: w246 -> [w249 w253]
                  frame #0 {
                    n231 = Index Array(array=w251, index=4) -> (element=w250:T6)
                    n232 = call "__move_motor2.vi"("Moving distance"=w249, "motor setup"=w250) -> ()  [unwired: 2 in, 2 out]
                  }
                  frame #1 {
                    n233 = Index Array(array=w255, index=5) -> (element=w254:T6)
                    n234 = call "__move_motor2.vi"("Moving distance"=w253, "motor setup"=w254) -> ()  [unwired: 2 in, 2 out]
                  }
                }
              }
            }
          }
          frame #8 {
            # "Vh2回目測定"
            n235 = flat-sequence {
              tunnel: [w287] -> w266
              tunnel: [w286] -> w262
              tunnel: [w285] -> w263
              frame #0 {
                n236 = while {
                  tunnel: [w275] -> _ mode=indexing
                  tunnel: [w274] -> _ mode=indexing
                  tunnel: [w273] -> _ mode=indexing
                  stop <- w278 stop-if-true
                  n237 = local read "初期時間（s）"() -> (w276:dbl)
                  n238 = local read "GC_LockinAmp"() -> (w272:T3)
                  n239 = Unbundle By Name(w272) -> ("wait(s)"=w283:dbl, "measure(s)"=w282:dbl)
                  n240 = expression code="4*x"(w283) -> (w281:dbl)
                  n241 = expression code="3*x"(w282) -> (w279:dbl)
                  n242 = Unbundle By Name(w272) -> ("GPIB"=w271:string)
                  n243 = Get Date/Time In Seconds() -> (seconds since 1Jan1904=w284:timestamp)
                  n244 = local read "TC"() -> (w270:dbl)
                  n245 = Compound Arithmetic op=ADD(w276, w281, w279) -> (w280:dbl)
                  n246 = To Double Precision Float(number=w284) -> (double precision float=w277:dbl)
                  n247 = Subtract(x=w277, y=w276) -> (x-y=w274:dbl)
                  n248 = Wait (ms)(milliseconds to wait=w270) -> ()  [unwired: 1 out]
                  n249 = call "__SR530_read.vi"("GPIB"=w271) -> ("Phase"=w273:dbl, "R"=w275:dbl)  [unwired: 5 in]
                  n250 = local write "経過時間（s）"(w274) -> ()
                  n251 = Greater?(x=w277, y=w280) -> (0:w278:bool)
                  n252 = local write "R"(w275) -> ()
                  n253 = local write "P"(w273) -> ()
                }
              }
              frame #1 {
                n254 = while {
                  tunnel: [w293] -> w286 mode=indexing
                  tunnel: [w292] -> w287 mode=indexing
                  tunnel: [w291] -> w285 mode=indexing
                  stop <- w296 stop-if-true
                  n255 = local read "初期時間（s）"() -> (w294:dbl)
                  n256 = local read "GC_LockinAmp"() -> (w290:T3)
                  n257 = Unbundle By Name(w290) -> ("wait(s)"=w301:dbl, "measure(s)"=w300:dbl)
                  n258 = expression code="4*x"(w301) -> (w299:dbl)
                  n259 = expression code="4*x"(w300) -> (w297:dbl)
                  n260 = Unbundle By Name(w290) -> ("GPIB"=w289:string)
                  n261 = Get Date/Time In Seconds() -> (seconds since 1Jan1904=w302:timestamp)
                  n262 = local read "TC"() -> (w288:dbl)
                  n263 = Compound Arithmetic op=ADD(w294, w299, w297) -> (w298:dbl)
                  n264 = To Double Precision Float(number=w302) -> (double precision float=w295:dbl)
                  n265 = Subtract(x=w295, y=w294) -> (x-y=w292:dbl)
                  n266 = Wait (ms)(milliseconds to wait=w288) -> ()  [unwired: 1 out]
                  n267 = call "__SR530_read.vi"("GPIB"=w289) -> ("Phase"=w291:dbl, "R"=w293:dbl)  [unwired: 5 in]
                  n268 = local write "経過時間（s）"(w292) -> ()
                  n269 = Greater?(x=w295, y=w298) -> (0:w296:bool)
                  n270 = local write "R"(w293) -> ()
                  n271 = local write "P"(w291) -> ()
                }
              }
            }
            n272 = local read "AR"() -> (w264:dbl[])
            n273 = local read "AP"() -> (w265:dbl[])
            n274 = local read "AT"() -> (w267:dbl[])
            n275 = call <vilib>:"Std Deviation and Variance.vi"("X"=w262) -> ("mean"=w269:dbl, "standard deviation"=w268:dbl)  [unwired: 1 in, 1 out]
            n276 = Insert Into Array(array=w264, new element=w262) -> (w259:dbl[])  [unwired: 1 in]
            n277 = Insert Into Array(array=w265, new element=w263) -> (w260:dbl[])  [unwired: 1 in]
            n278 = Insert Into Array(array=w267, new element=w266) -> (w261:dbl[])  [unwired: 1 in]
            n279 = local write "Vh2 σ"(w268) -> ()
            n280 = local write "Vh2"(w269) -> ()
            n281 = local write "AR"(w259) -> ()
            n282 = local write "AP"(w260) -> ()
            n283 = local write "AT"(w261) -> ()
            n284 = Bundle("AT"=w261, "AP"=w260) -> (w257:cluster{"AT":dbl[], "AP":dbl[]})  [unwired: 1 in]
            n285 = Bundle("AT"=w261, "AR"=w259) -> (w258:cluster{"AT":dbl[], "AR ":dbl[]})  [unwired: 1 in]
            n286 = local write "XYグラフ 2"(w257) -> ()
            n287 = local write "XYグラフ"(w258) -> ()
          }
          frame #9 {
            # "モーター Cold"
            n288 = local read "Control"() -> (w303:T4)
            n289 = Unbundle By Name(w303) -> ("HOT/COLD"=w304:u16)
            n290 = case shown="0, 기본" w304 {
              tunnel: w303 -> [w309 w313 w324]
              tunnel: -50.0 -> [w306 w311 w322]
              frame 0, Default {
                n291 = Unbundle By Name(w309) -> ("mortor設定"=w308:T5)
                n292 = Index Array(array=w308, index=0) -> (element=w307:T6)
                n293 = call "__move_motor2.vi"("Moving distance"=w306, "motor setup"=w307) -> ()  [unwired: 2 in, 2 out]
              }
              frame 1 {
                n294 = Unbundle By Name(w313) -> ("mortor設定"=w312:T5)
                n295 = stacked-sequence {
                  tunnel: w312 -> [w316 w320]
                  tunnel: w311 -> [w314 w318]
                  frame #0 {
                    n296 = Index Array(array=w316, index=2) -> (element=w315:T6)
                    n297 = call "__move_motor2.vi"("Moving distance"=w314, "motor setup"=w315) -> ()  [unwired: 2 in, 2 out]
                  }
                  frame #1 {
                    n298 = Index Array(array=w320, index=3) -> (element=w319:T6)
                    n299 = call "__move_motor2.vi"("Moving distance"=w318, "motor setup"=w319) -> ()  [unwired: 2 in, 2 out]
                  }
                }
              }
              frame 2 {
                n300 = Unbundle By Name(w324) -> ("mortor設定"=w323:T5)
                n301 = stacked-sequence {
                  tunnel: w323 -> [w327 w331]
                  tunnel: w322 -> [w325 w329]
                  frame #0 {
                    n302 = Index Array(array=w327, index=4) -> (element=w326:T6)
                    n303 = call "__move_motor2.vi"("Moving distance"=w325, "motor setup"=w326) -> ()  [unwired: 2 in, 2 out]
                  }
                  frame #1 {
                    n304 = Index Array(array=w331, index=5) -> (element=w330:T6)
                    n305 = call "__move_motor2.vi"("Moving distance"=w329, "motor setup"=w330) -> ()  [unwired: 2 in, 2 out]
                  }
                }
              }
            }
          }
          frame #10 {
            w339 = 0.8
            w340 = 1.5
            n306 = local read "Vh1 σ"() -> (w345:dbl)
            n307 = local read "Vh2 σ"() -> (w344:dbl)
            n308 = local read "Vc2 σ"() -> (w341:dbl)
            n309 = local read "Vh2"() -> (w352:dbl)
            n310 = local read "Vc2"() -> (w354:dbl)
            n311 = local read "Vc1 σ"() -> (w337:dbl)
            n312 = local read "Vh1"() -> (w353:dbl)
            n313 = local read "Vc1"() -> (w355:dbl)
            n314 = Divide(x=w345, y=w344) -> (x/y=w343:dbl)
            n315 = In Range and Coerce(upper limit=w340, x=w343, lower limit=w339) -> (In Range?=w334:bool)  [unwired: 1 out]
            "Vh σ" <- w334
            n316 = Divide(x=w337, y=w341) -> (x/y=w342:dbl)
            n317 = In Range and Coerce(upper limit=w340, x=w342, lower limit=w339) -> (In Range?=w333:bool)  [unwired: 1 out]
            "Ｖｃ　σ" <- w333
            n318 = expression code="3*x"(w345) -> (w349:dbl)
            n319 = expression code="3*x"(w337) -> (w351:dbl)
            n320 = Subtract(x=w355, y=w354) -> (x-y=w350:dbl)
            n321 = formula code="float gcls,gc,E;\ngc=(vc-vh)/vc*100;\ngcls=gc/2*1.2793+0.11;\nE=gcls*3*sigma/vc;"("vc"=w354, "vh"=w352, "sigma"=w341) -> ("gcls"=→"GCls  2":dbl, "gc"=→"GCdiff 2":dbl, "E"=→"Error 2":dbl)
            n322 = Subtract(x=w353, y=w352) -> (x-y=w348:dbl)
            n323 = formula code="float gcls,gc,E;\ngc=(vc-vh)/vc*100;\ngcls=gc/2*1.2793+0.11;\nE=gcls*3*sigma/vc;"("vc"=w355, "vh"=w353, "sigma"=w337) -> ("gcls"=→"GCls  1":dbl, "gc"=→"GCdiff 1":dbl, "E"=→"Error 1":dbl)
            n324 = Absolute Value(x=w350) -> (abs(x)=w347:dbl)
            "ΔVc" <- w347
            n325 = Absolute Value(x=w348) -> (abs(x)=w346:dbl)
            "ΔVh" <- w346
            n326 = Greater?(x=w349, y=w346) -> (0:w335:bool)
            "Vh" <- w335
            n327 = Greater?(x=w351, y=w347) -> (0:w336:bool)
            "Vc" <- w336
            n328 = Compound Arithmetic op=AND(w336, w335, w334, w333) -> (w338:bool)
          }
        }
        n329 = Greater?(x=3, y=w5) -> (0:w8:bool)
        n330 = Not(x=w8) -> (.not. x?=w6:bool)
        n331 = Or(x=w9, y=w6) -> (x .or. y?=w7:bool)
        "測定回数" <- w5
      }
    }
    frame #1 {
      n332 = local read "Vc1 σ"() -> (w368:dbl)
      n333 = local read "GCls  1"() -> (w378:dbl)
      n334 = local read "GCls  2"() -> (w377:dbl)
      n335 = local read "Vh1"() -> (w369:dbl)
      n336 = local read "Vc1"() -> (w370:dbl)
      n337 = local read "Bias_LO_equip"() -> (w379:T1)
      n338 = local read "Control"() -> (w382:T4)
      n339 = local read "GCdiff 1"() -> (w367:dbl)
      n340 = local read "GCls  1"() -> (w366:dbl)
      n341 = Add(x=w378, y=w377) -> (x+y=w376:dbl)
      n342 = Get Date/Time In Seconds() -> (seconds since 1Jan1904=w381:timestamp)
      n343 = expression code="x/2"(w376) -> (w371:dbl)
      n344 = Unbundle By Name(w382) -> ("FreqLO"=w373:dbl)
      n345 = Unbundle By Name(w379) -> ("POL"=w372:u32)
      n346 = Format Date/Time String(time format string (%c)="%Y-%m-%d  %H:%M:%S", seconds (now)=w381) -> (date/time string=w374:string)  [unwired: 1 in]
      n347 = Format Into String(format string="GainComp, %s, %.2f,%d, 0, %2.2f,, %.3e, %.3e, %.3e, %.3e, %.3e", w374, w373, w372, w371, w370, w369, w368, w367, w366) -> (resulting string=w363:string)  [unwired: 2 in, 1 out]
      n348 = local write "出力文字列"(w363) -> ()
      n349 = local read "GC_LockinAmp"() -> (w365:T3)
      n350 = Unbundle By Name(w365) -> ("save"=w364:bool, "file_name"=w362:string)
      n351 = case shown="참" w364 {
        tunnel: w363 -> [_ w390]
        tunnel: w362 -> [_ w389]
        frame False {
        }
        frame True {
          n352 = local read "AR"() -> (w386:dbl[])
          n353 = local read "Control"() -> (w393:T4)
          n354 = local read "AT"() -> (w385:dbl[])
          n355 = local read "AP"() -> (w387:dbl[])
          n356 = Unbundle By Name(w393) -> ("DATAパス"=w383:path)
          n357 = Build Array(w385, w386, w387) -> (w384:dbl[][])
          n358 = Format Into String(format string="%s \\n Time,R,P", w390) -> (resulting string=w388:string)  [unwired: 2 in, 1 out]
          n359 = call "___save_2d_data_with_header.vi"("ヘッダー"=w388, "配列"=w384, "形式"="%^.3e", "file_name"=w389, "パス"=w383) -> ()  [unwired: 6 in, 1 out]
        }
      }
    }
  }
